vi "AG34980A_Configure_Trigger.vi"(0 "VISA resource name":refnum<visa-resource-name>, 1 "Trigger Timer Value (0 sec)":dbl max=359999.0 format="%#_2e", 2 "Sample Count (1)":u32=1 min=1 max=500000 step=1, 5 "Trigger Source (1:Immediate)":T1(ring)=enum."Immediate", 7 "Max Trigger Count (0:Specify Count)":enum16{"Specify Count", "Infinity"}(ring), 9 "# Triggers (1)":u32=1 max=500000 step=1, 11 "error in (no error)":errorcluster, 12 "Trigger Delay (0 sec)":dbl, 13 "Trigger Delay Auto? (T:On)":bool=TRUE) -> (4 "VISA resource name out":refnum<visa-resource-name>, 15 "error out":errorcluster)   [LabVIEW 2022 SP3, in "DMM_Keysight_34980A.lvlib" / "DMM_Keysight_34980A.lvclass"]
doc: "This VI allows you to specify various settings for controlling the triggering system. You can independently specify the trigger source and trigger count, as well as the time-scan interval and trigger delay."
uses:
  DMM_Keysight_34980A.lvclass
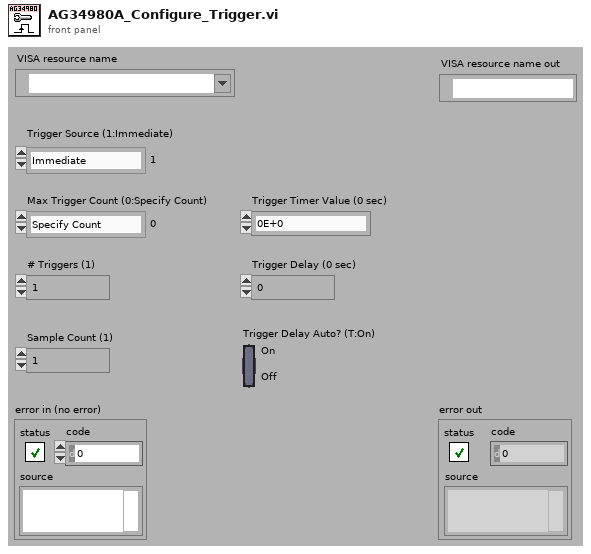
[diagram p1: front panel]
types:
  T1 = enum16{"Bus", "Immediate", "External", "Alarm 1", "Alarm 2", "Alarm 3", "Alarm 4", "Timer"}
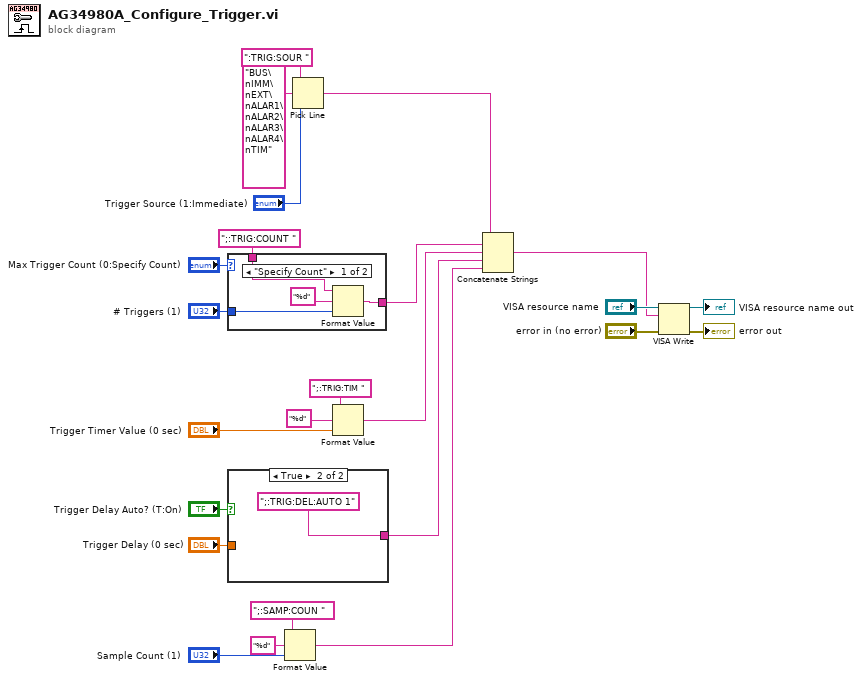
[diagram p0: block diagram]
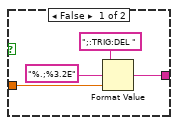
[diagram p2: hidden frame]
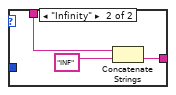
[diagram p3: hidden frame]
diagram:
  n1 = case shown="\"Specify Count\"" "Max Trigger Count (0:Specify Count)" {
    tunnel: ";:TRIG:COUNT " -> [w27 w30]
    tunnel: [w26 w29] -> w11
    tunnel: "# Triggers (1)" -> [w25 _]
    frame "Specify Count" {
      n2 = Format Value(string ("")=w27, format string="%d", value (0)=w25) -> (output string=w26:string)
    }
    frame "Infinity" {
      n3 = Concatenate Strings(w30, "INF") -> (w29:string)
    }
  }
  n4 = case shown="True" "Trigger Delay Auto? (T:On)" {
    tunnel: "Trigger Delay (0 sec)" -> [w33 _]
    tunnel: [w32 ";:TRIG:DEL:AUTO 1"] -> w7
    frame False {
      n5 = Format Value(string ("")=";:TRIG:DEL ", format string="%.;%3.2E", value (0)=w33) -> (output string=w32:string)
    }
    frame True {
    }
  }
  n6 = Format Value(string ("")=";:SAMP:COUN ", format string="%d", value (0)="Sample Count (1)") -> (output string=w3:string)
  n7 = Pick Line(string ("")=":TRIG:SOUR ", multi-line string="BUS\nIMM\nEXT\nALAR1\nALAR2\nALAR3\nALAR4\nTIM", line index="Trigger Source (1:Immediate)") -> (output string=w12:string)
  n8 = Format Value(string ("")=";:TRIG:TIM ", format string="%d", value (0)="Trigger Timer Value (0 sec)") -> (output string=w10:string)
  n9 = Concatenate Strings(w12, w11, w10, w7, w3) -> (w6:string)
  n10 = VISA Write(VISA resource name="VISA resource name", write buffer=w6, error in (no error)="error in (no error)") -> (VISA resource name out=→"VISA resource name out":refnum<visa-resource-name>, error out=→"error out":errorcluster)  [unwired: 1 out]
